vi "ziGetEventDoubleDataTS.vi"(8 "Error In":errorcluster, 10 "Sample In":T1, 11 "Handle In":T2 {"Handle" format="0x%08x"; "Conn" format="0x%08x"}) -> (0 "Error Out":errorcluster, 2 "Sample Out":T1, 3 "Handle Out":T2 {"Handle" format="0x%08x"; "Conn" format="0x%08x"})   [LabVIEW 2009, in "Zurich Instruments LabOne.lvlib"]
uses:
  <instrlib>/Zurich Instruments LabOne/Zurich Instruments LabOne.lvlib
  <instrlib>/Zurich Instruments LabOne/Public/ziTypeHandle.ctl
  <instrlib>/Zurich Instruments LabOne/Public/Data/ziTypeDoubleDataTS.ctl
  <instrlib>/Zurich Instruments LabOne/Private/ziLV32.dll
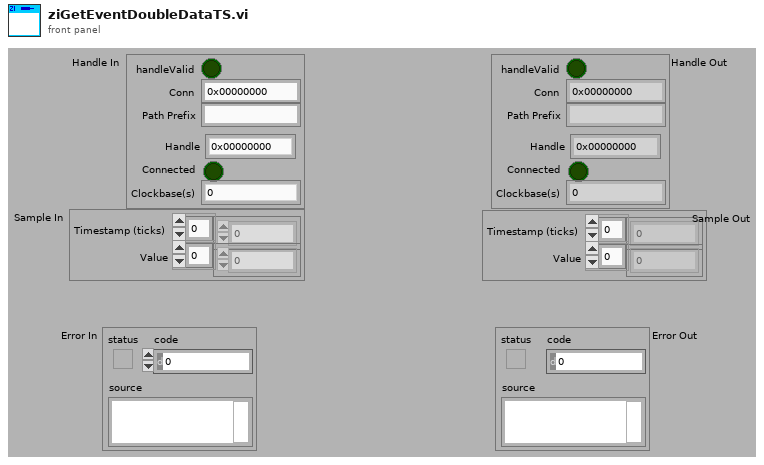
[diagram p1: front panel]
types:
  T1 = typedef "Zurich Instruments LabOne.lvlib/ziTypeDoubleDataTS.ctl" = cluster{"Timestamp (ticks)":u64[], "Value":dbl[]}
  T2 = typedef "Zurich Instruments LabOne.lvlib/ziTypeHandle.ctl" = cluster{"handleValid":bool, "Conn":u64, "Path Prefix":string, "Handle":u64, "Connected":bool, "Clockbase(s)":dbl}
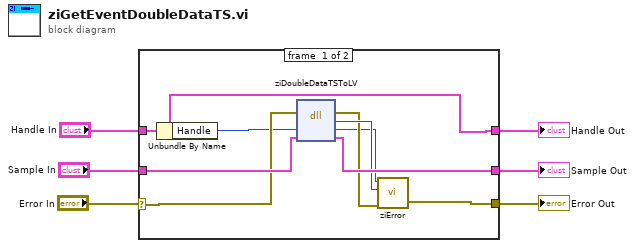
[diagram p0: block diagram]
diagram:
  n1 = case shown="No Error" "Error In" {
    selector: "Error In" -> [w13 w18]
    tunnel: "Handle In" -> [w8 w16]
    tunnel: [w8 w16] -> w5
    tunnel: [w15 w17] -> w4
    tunnel: "Sample In" -> [w14 w17]
    tunnel: [w12 w18] -> w2
    frame #0 {
      n2 = Unbundle By Name(w8) -> ("Handle"=w11:u64)
      n3 = dll-call lib="C:/Program Files (x86)/National Instruments/LabVIEW 2009/instr.lib/Zurich Instruments LabOne/Private/ziLV*.*" fn="ziDoubleDataTSToLV"(error in=w13, "ziEventBuffer"=w11, "DoubleSample"=w14) -> (error out=w9:errorcluster, "return type"=w10:u32, "ziEventBuffer"=w7:u64, "DoubleSample"=w15:T1)  [unwired: 2 in, 1 out]
      n4 = call <instrlib>:"ziError.vi"("Conn"=w7, "ziErrorCode"=w10, "Error In"=w9) -> ("Error Out"=w12:errorcluster)  [unwired: 2 in, 1 out]
    }
    frame #1 {
    }
  }
  "Handle Out" <- w5
  "Sample Out" <- w4
  "Error Out" <- w2
